vi "input limits.vi"(5 "Server Method":T1={"scan rate (Hz)"=100.0, "Channel group array"=[], "Number of groups"=1} {"Number of groups" min=1; "Channel group array"."max voltage" format="%.4f"; "scan rate (Hz)" format="%.2f"}) -> (2 "input limits (no change)":cluster{"high limit":sgl, "low limit":sgl}[](array[cluster]) {"low limit" format="%.2f"; "high limit" format="%.3f"})   [LabVIEW 2010]
uses:
  Dataserver method.ctl
panel:
  # "Hz"
  # "channel identifiers"
  # "max voltage"
  # "port locations"
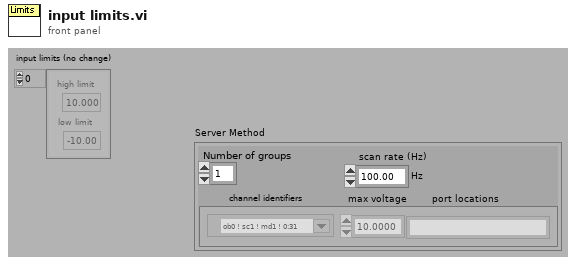
[diagram p1: front panel]
types:
  T1 = typedef "Dataserver method.ctl" = cluster{"scan rate (Hz)":dbl, "Channel group array":cluster{"channels":tag, "max voltage":sgl, "Port locations":string}[], "Number of groups":u8}
  T2 = cluster{"channels":tag, "max voltage":sgl, "Port locations":string}[]
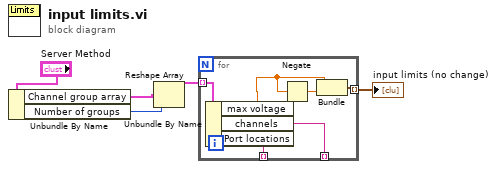
[diagram p0: block diagram]
diagram:
  n1 = Unbundle By Name("Server Method") -> ("Channel group array"=w2:T2, "Number of groups"=w1:u8)
  n2 = Reshape Array(w2, w1) -> (w5:T2)
  n3 = for {
    tunnel: w5 -> [w10] mode=indexing
    tunnel: [w11] -> w4 mode=indexing
    tunnel: [w9] -> _ mode=indexing
    tunnel: [w8] -> _ mode=indexing
    n4 = Unbundle By Name(w10) -> ("max voltage"=w6:sgl, "channels"=w9:tag, "Port locations"=w8:string)
    n5 = Negate(x=w6) -> (-x=w7:sgl)
    n6 = Bundle("max voltage"=w6, w7) -> (w11:cluster{"max voltage":sgl, sgl})  [unwired: 1 in]
  }
  "input limits (no change)" <- w4
